vi "Read debug cluster.vi"() -> ()   [LabVIEW 2021]
uses:
  Driver/SubVIS/CANOpen_Settings.ctl
  Driver/SubVIS/CANOpen_Node Settings.ctl
  Shared Code/CANOpen_Bus Settings.ctl
  Shared Code/CANOpen Interface Name.ctl
  <vilib>/CANopenLib/CANOPEN.llb/CANopen BaudRate.ctl
  Driver/SubVIS/CANOpen_Node Message Settings.ctl
  Shared Code/CANOpen_PDO Settings.ctl
  Shared Code/CANOpen_PDO Parameter Settings.ctl
  Shared Code/CANOpen_PDO Data Type.ctl
  System Explorer/SubVIs/CANopen Byte Order.ctl
  Shared Code/CANOpen_SDO Settings.ctl
  Driver/SubVIS/CANOpen_NMT Settings.ctl
  Driver/Async VIs/CANOpen_Main/SubVIs/CanOpen_NMT_Config.ctl
  Driver/Async VIs/CANOpen_Main/SubVIs/CanOpen_NMT_Static detect.ctl
  Driver/Async VIs/CANOpen_Main/SubVIs/CanOpen_Main Node Ids.ctl
  Driver/SubVIS/CANOpen_VS Data Refs.ctl
  <vilib>/NI VeriStand/Custom Device API/Data Reference.ctl
  <vilib>/NI VeriStand/Custom Device API/Block Data Reference.ctl
  Driver/SubVIS/CANOpen_VS Bidirectional Data Refs.ctl
  Driver/SubVIS/CANOpen_VS SDOs Data Refs.ctl
  Driver/Async VIs/CANOpen_Main/SubVIs/CanOpen_SDO Dynamic queue.ctl
  Shared Code/CANOpen_SDO queue W data.ctl
  Shared Code/CANOpen_SDO queue mode.ctl
  Shared Code/CANOpen_PDO Data Type in queue.ctl
  Driver/SubVIS/CANOpen_VS Status Management Data Refs.ctl
  Driver/Async VIs/CANOpen_Main/SubVIs/CanOpen_NMT_HWOut_ChannelPairs.ctl
  Driver/Async VIs/CANOpen_Main/SubVIs/CanOpen_NMT_HWIn_ChannelPairs.ctl
  SubVIs/Global debug.vi
  <vilib>/NI VeriStand/Custom Device API/Custom Device API.lvlib
panel:
  out "Configuration Cluster":T1={"Driver Settings"={"CANOpen Bus Settings"={"CANOpen Interface Name"=0, "Baud Rate"=0, "Termination"=FALSE, "Sync Period (ms)"=10, "Enable 9881"=FALSE, "RIO Device"=0, "Enable SYNC"=FALSE, "Scan & Print"=FALSE}, "Nodes"=[], "Node Ids"=[]}, "Data References"={"Hardware Input"={"FIFO"=refnum, "Channel Pairs"={"Chan Refs"=[], "Prev. Values"=[]}}, "Hardware Output"={"FIFO"=refnum, "Channel Pairs"={"Block Refs"=[], "Prev. Values"=[]}}}, "Bus Commands"={"Hardware Output"={"FIFO"=refnum, "Channel Pairs"={"Chan Refs"=[], "Prev. Values"=[]}}, "Hardware Input"={"FIFO"=refnum}}, "SDO Asynch"={"List SDO"={"FIFO Req"=refnum, "Req Chan."={"Chan Refs"=[], "NodeIndex"=[]}, "FIFO Resp"=refnum, "Resp Chan."={"Chan Refs"=[]}, "Node IDs"=[], "FIFO array"=[]}, "HW Dyn Write"={"FIFO Req"=refnum, "FIFO Resp"=refnum, "Req Chan."={"Chan Refs"=[], "Node IDs"=[]}, "Resp Chan."={"Chan Refs"=[]}}, "HW Dyn Read"={"FIFO Req"=refnum, "FIFO Resp"=refnum, "Req Chan."={"Chan Refs"=[], "Node IDs"=[]}, "Resp Chan."={"Chan Refs"=[]}}}, "Status NMT"={"Hardware Output"={"FIFO"=refnum, "Channel Pairs"={"Chan Refs"=[], "Prev. Values"=[], "Node index"=[]}}, "Hardware Input"={"FIFO"=refnum, "Channel Pairs"={"Chan Refs"=[], "Prev. Values"=[], "Node index"=[]}}}} {"Status NMT"."Hardware Output"."Channel Pairs"."Chan Refs"."Data Reference" format="%.0x"; "Status NMT"."Hardware Input"."Channel Pairs"."Chan Refs" format="%.0x"; "SDO Asynch"."HW Dyn Read"."Resp Chan."."Chan Refs" format="%.0x"; "SDO Asynch"."HW Dyn Read"."Req Chan."."Chan Refs" format="%.0x"; "SDO Asynch"."HW Dyn Write"."Resp Chan."."Chan Refs" format="%.0x"; "SDO Asynch"."HW Dyn Write"."Req Chan."."Chan Refs" format="%.0x"; "SDO Asynch"."List SDO"."Resp Chan."."Chan Refs" format="%.0x"; "SDO Asynch"."List SDO"."Req Chan."."Chan Refs" format="%.0x"; "Bus Commands"."Hardware Output"."Channel Pairs"."Chan Refs" format="%.0x"; "Data References"."Hardware Input"."Channel Pairs"."Chan Refs" format="%.0x"; "Data References"."Hardware Output"."Channel Pairs"."Block Refs"."Data Reference" format="%.0x"; "Driver Settings"."CANOpen Bus Settings"."Baud Rate" items=["1 Mbit/s"=0, "800 kbit/s"=1, "500 kbit/s"=2, "250 kbit/s"=3, "125 kbit/s"=4, "50 kbit/s"=6, "20 kbit/s"=7, "10 kbit/s"=8]; "Driver Settings"."CANOpen Bus Settings"."CANOpen Interface Name" items=["CANopen01", "CANopen02", "CANopen03", "CANopen04", "CANopen05", "CANopen06", "CANopen07", "CANopen08", "CANopen09", "CANopen10", "CANopen11", "CANopen12", "CANopen13", "CANopen14", "CANopen15", "CANopen16", "CANopen17", "CANopen18", "CANopen19", "CANopen20", "CANopen21", "CANopen22", "CANopen23", "CANopen24", "CANopen25", "CANopen26", "CANopen27", "CANopen28", "CANopen29", "CANopen30", "CANopen31", "CANopen32"]; "Driver Settings"."Nodes"."NMT"."Node init static SDO state" items=["start remote node"=1, "enter pre-operational"=128]; "Driver Settings"."Nodes"."NMT"."Node run state" items=["start remote node"=1, "stop remote node"=2, "enter pre-operational"=128, "reset node"=129, "reset communication"=130]; "Driver Settings"."Nodes"."Dynamic SDOs"."Sub-Index (0)" format="%.0x"; "Driver Settings"."Nodes"."Dynamic SDOs"."Object Index" format="%.0x"; "Driver Settings"."Nodes"."Dynamic SDOs"."Block Data" format="%.0x"; "Driver Settings"."Nodes"."RPDOs"."PDO Channel" items=["PDO 1", "PDO 2", "PDO 3", "PDO 4"]; "Driver Settings"."Nodes"."TPDOs"."PDO Channel" items=["PDO 1", "PDO 2", "PDO 3", "PDO 4"]; "Driver Settings"."Nodes"."SDOs"."Sub-Index (0)" format="%.0x"; "Driver Settings"."Nodes"."SDOs"."Object Index" format="%.0x"; "Driver Settings"."Nodes"."SDOs"."Block Data" format="%.0x"}
  # "LSB"
  # "MSB"
  # "LSB"
  # "MSB"
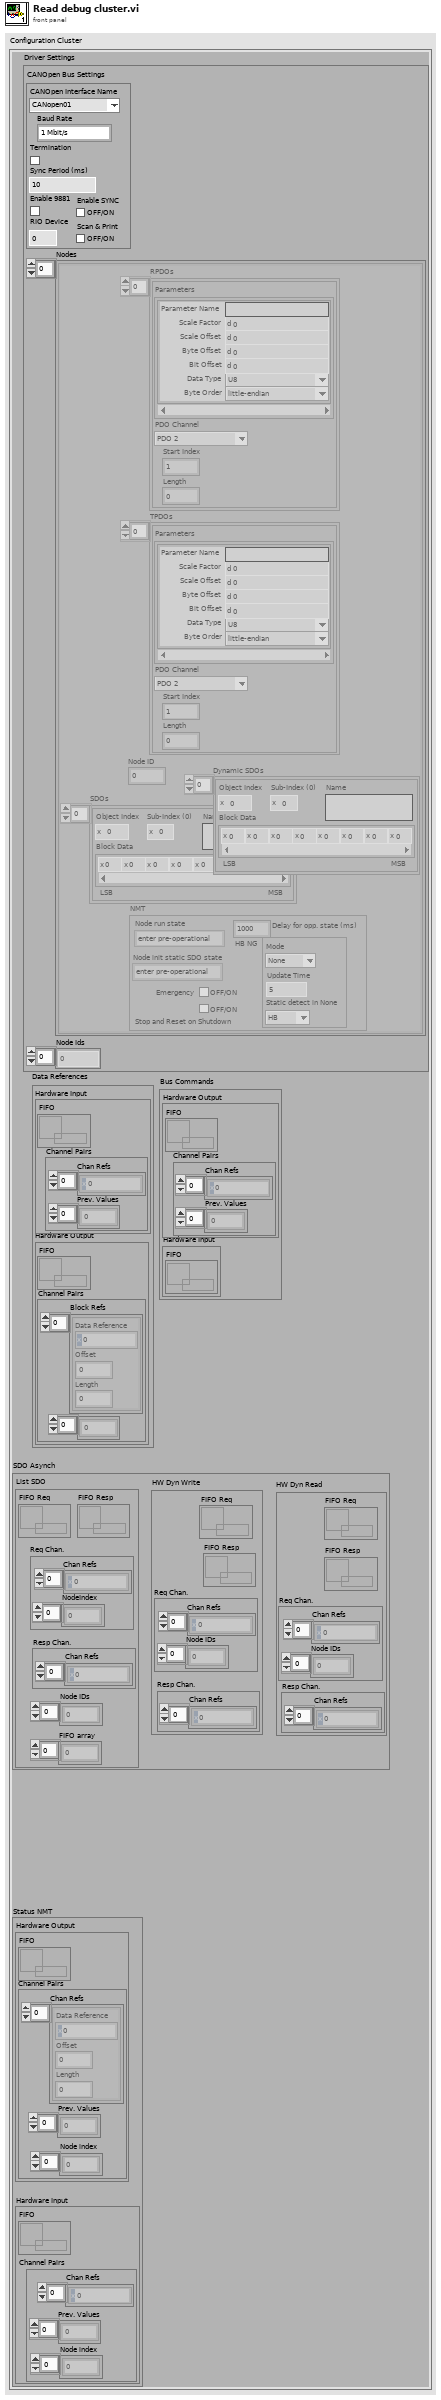
[diagram p1: front panel]
types:
  T1 = typedef "CANOpen_Settings.ctl" = cluster{"Driver Settings":T2, "Data References":T16, "Bus Commands":T19, "SDO Asynch":T20, "Status NMT":T21}
  T2 = typedef "CANOpen_Node Settings.ctl" = cluster{"CANOpen Bus Settings":T3, "Nodes":T6[], "Node Ids":T15}
  T3 = typedef "CANOpen_Bus Settings.ctl" = cluster{"CANOpen Interface Name":T4, "Baud Rate":T5, "Termination":bool, "Sync Period (ms)":i64, "Enable 9881":bool, "RIO Device":u16, "Enable SYNC":bool, "Scan & Print":bool}
  T4 = typedef "CANOpen Interface Name.ctl" = u32
  T5 = typedef "CANopen BaudRate.ctl" = u32
  T6 = typedef "CANOpen_Node Message Settings.ctl" = cluster{"RPDOs":T7[], "TPDOs":T7[], "Node ID":u8, "SDOs":T11[], "Dynamic SDOs":T11[], "NMT":T12}
  T7 = typedef "CANOpen_PDO Settings.ctl" = cluster{"Parameters":T8[], "PDO Channel":u8, "Start Index":u32, "Length":u32}
  T8 = typedef "CANOpen_PDO Parameter Settings.ctl" = cluster{"Parameter Name":string, "Scale Factor":dbl, "Scale Offset":dbl, "Byte Offset":u8, "Bit Offset":u8, "Data Type":T9, "Byte Order":T10}
  T9 = typedef "CANOpen_PDO Data Type.ctl" = enum16{"U8", "U16", "U32", "I8", "I16", "I32", "Single", "Double", "Boolean"}
  T10 = typedef "CANopen Byte Order.ctl" = enum16{"big-endian network order", "little-endian"}
  T11 = typedef "CANOpen_SDO Settings.ctl" = cluster{"Object Index":u16, "Sub-Index (0)":u8, "Block Data":u8[], "Name":string}
  T12 = typedef "CANOpen_NMT Settings.ctl" = cluster{"Node run state":u16, "Emergency":bool, "HB NG":T13, "Delay for opp. state (ms)":dbl, "Node init static SDO state":u16, "Stop and Reset on Shutdown":bool}
  T13 = typedef "CanOpen_NMT_Config.ctl" = cluster{"Mode":T14, "Update Time":u16, "Static detect in None":T14}
  T14 = typedef "CanOpen_NMT_Static detect.ctl" = enum16{"None", "HB", "NG"}
  T15 = typedef "CanOpen_Main Node Ids.ctl" = u8[]
  T16 = typedef "CANOpen_VS Data Refs.ctl" = cluster{"Hardware Input":cluster{"FIFO":refnum<k33>, "Channel Pairs":cluster{"Chan Refs":T17[], "Prev. Values":dbl[]}}, "Hardware Output":cluster{"FIFO":refnum<k33>, "Channel Pairs":cluster{"Block Refs":T18[], "Prev. Values":dbl[]}}}
  T17 = typedef "Custom Device API.lvlib/Data Reference.ctl" = i32
  T18 = typedef "Custom Device API.lvlib/Block Data Reference.ctl" = cluster{"Data Reference":T17, "Offset":u64, "Length":u64}
  T19 = typedef "CANOpen_VS Bidirectional Data Refs.ctl" = cluster{"Hardware Output":cluster{"FIFO":refnum<k33>, "Channel Pairs":cluster{"Chan Refs":T17[], "Prev. Values":dbl[]}}, "Hardware Input":cluster{"FIFO":refnum<k33>}}
  T20 = typedef "CANOpen_VS SDOs Data Refs.ctl" = cluster{"List SDO":cluster{"FIFO Req":refnum<k33>, "Req Chan.":cluster{"Chan Refs":T17[], "NodeIndex":dbl[]}, "FIFO Resp":refnum<k33>, "Resp Chan.":cluster{"Chan Refs":T17[]}, "Node IDs":u8[], "FIFO array":dbl[]}, "HW Dyn Write":cluster{"FIFO Req":refnum<k33>, "FIFO Resp":refnum<k33>, "Req Chan.":cluster{"Chan Refs":T17[], "Node IDs":u8[]}, "Resp Chan.":cluster{"Chan Refs":T17[]}}, "HW Dyn Read":cluster{"FIFO Req":refnum<k33>, "FIFO Resp":refnum<k33>, "Req Chan.":cluster{"Chan Refs":T17[], "Node IDs":u8[]}, "Resp Chan.":cluster{"Chan Refs":T17[]}}}
  T21 = typedef "CANOpen_VS Status Management Data Refs.ctl" = cluster{"Hardware Output":cluster{"FIFO":refnum<k33>, "Channel Pairs":T22}, "Hardware Input":cluster{"FIFO":refnum<k33>, "Channel Pairs":T23}}
  T22 = typedef "CanOpen_NMT_HWOut_ChannelPairs.ctl" = cluster{"Chan Refs":T18[], "Prev. Values":dbl[], "Node index":dbl[]}
  T23 = typedef "CanOpen_NMT_HWIn_ChannelPairs.ctl" = cluster{"Chan Refs":T17[], "Prev. Values":dbl[], "Node index":dbl[]}
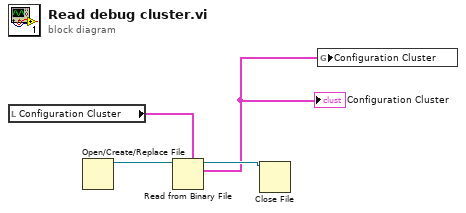
[diagram p0: block diagram]
diagram:
  n1 = local read "Configuration Cluster"() -> (w3:T1)
  n2 = Open/Create/Replace File() -> (refnum out=w4:refnum<file>)  [unwired: 6 in, 2 out]
  n3 = Read from Binary File(5:w3, 11:w4) -> (2:w1:T1, 3:w2:refnum<file>)  [unwired: 4 in, 2 out]
  "Configuration Cluster" <- w1
  n4 = Close File(refnum=w2) -> ()  [unwired: 1 in, 2 out]
  n5 = global write "Global debug.vi" "Configuration Cluster"(w1) -> ()
